vi "10-2.vi"() -> ()   [LabVIEW 2022 SP3, in "AoC22.lvlib"]
uses:
  AoC22.lvlib
  <vilib>/IlluminatedG/lv-stream/Stream.lvlib
panel:
  out "Array":bool[][](array[boolean])
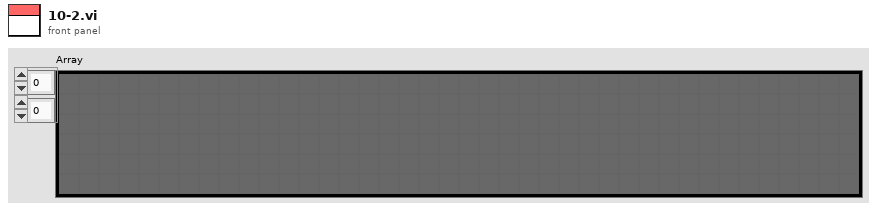
[diagram p1: front panel]
types:
  T1 = cluster{"String":string, "String":string, "x":i32, i32, i32, bool}
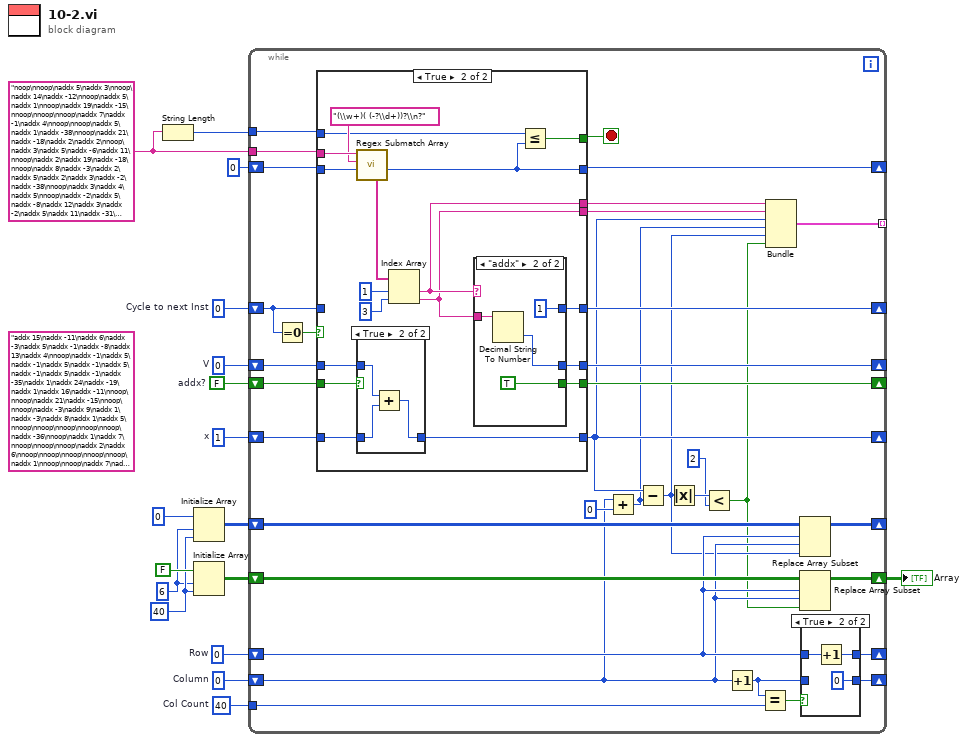
[diagram p0: block diagram]
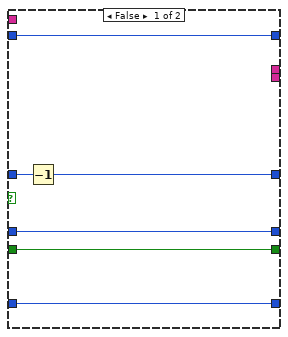
[diagram p3: hidden frame]
diagram:
  w4 = 40 ("dimension size")
  w3 = 6 ("dimension size")
  w9 = 0  # Row
  (unwired) "addx 15\naddx -11\naddx 6\naddx -3\naddx 5\naddx -1\naddx -8\naddx 13\naddx 4\nnoop\naddx -1\naddx 5\naddx -1\naddx 5\naddx -1\naddx 5\naddx -1\naddx 5\naddx -1\naddx -35\naddx 1\naddx 24\naddx -19\naddx 1\naddx 16\naddx -11\nnoop\nnoop\naddx 21\naddx -15\nnoop\nnoop\naddx -3\naddx 9\naddx 1\naddx -3\naddx 8\naddx 1\naddx 5\nnoop\nnoop\nnoop\nnoop\nnoop\naddx -36\nnoop\naddx 1\naddx 7\nnoop\nnoop\nnoop\naddx 2\naddx 6\nnoop\nnoop\nnoop\nnoop\nnoop\naddx 1\nnoop\nnoop\naddx 7\naddx 1\nnoop\naddx -13\naddx 13\naddx 7\nnoop\naddx 1\naddx -33\nnoop\nnoop\nnoop\naddx 2\nnoop\nnoop\nnoop\naddx 8\nnoop\naddx -1\naddx 2\naddx 1\nnoop\naddx 17\naddx -9\naddx 1\naddx 1\naddx -3\naddx 11\nnoop\nnoop\naddx 1\nnoop\naddx 1\nnoop\nnoop\naddx -13\naddx -19\naddx 1\naddx 3\naddx 26\naddx -30\naddx 12\naddx -1\naddx 3\naddx 1\nnoop\nnoop\nnoop\naddx -9\naddx 18\naddx 1\naddx 2\nnoop\nnoop\naddx 9\nnoop\nnoop\nnoop\naddx -1\naddx 2\naddx -37\naddx 1\naddx 3\nnoop\naddx 15\naddx -21\naddx 22\naddx -6\naddx 1\nnoop\naddx 2\naddx 1\nnoop\naddx -10\nnoop\nnoop\naddx 20\naddx 1\naddx 2\naddx 2\naddx -6\naddx -11\nnoop\nnoop\nnoop"
  w11 = 40  # Col Count
  w12 = 0  # Column
  w13 = FALSE  # addx?
  w15 = 1  # x
  w14 = 0  # V
  w16 = 0  # Cycle to next Inst
  w1 = "noop\nnoop\naddx 5\naddx 3\nnoop\naddx 14\naddx -12\nnoop\naddx 5\naddx 1\nnoop\naddx 19\naddx -15\nnoop\nnoop\nnoop\naddx 7\naddx -1\naddx 4\nnoop\nnoop\naddx 5\naddx 1\naddx -38\nnoop\naddx 21\naddx -18\naddx 2\naddx 2\nnoop\naddx 3\naddx 5\naddx -6\naddx 11\nnoop\naddx 2\naddx 19\naddx -18\nnoop\naddx 8\naddx -3\naddx 2\naddx 5\naddx 2\naddx 3\naddx -2\naddx -38\nnoop\naddx 3\naddx 4\naddx 5\nnoop\naddx -2\naddx 5\naddx -8\naddx 12\naddx 3\naddx -2\naddx 5\naddx 11\naddx -31\naddx 23\naddx 4\nnoop\nnoop\naddx 5\naddx 3\naddx -2\naddx -37\naddx 1\naddx 5\naddx 2\naddx 12\naddx -10\naddx 3\naddx 4\naddx -2\nnoop\naddx 6\naddx 1\nnoop\nnoop\nnoop\naddx -2\naddx 7\naddx 2\nnoop\naddx 3\naddx 3\naddx 1\nnoop\naddx -37\naddx 2\naddx 5\naddx 2\naddx 32\naddx -31\naddx 5\naddx 2\naddx 9\naddx 9\naddx -15\nnoop\naddx 3\naddx 2\naddx 5\naddx 2\naddx 3\naddx -2\naddx 2\naddx 2\naddx -37\naddx 5\naddx -2\naddx 2\naddx 5\naddx 2\naddx 16\naddx -15\naddx 4\nnoop\naddx 1\naddx 2\nnoop\naddx 3\naddx 5\naddx -1\naddx 5\nnoop\nnoop\nnoop\nnoop\naddx 3\naddx 5\naddx -16\nnoop"
  n1 = String Length(string=w1) -> (length=w17:i32)
  n2 = Initialize Array(0, w3, w4) -> (w2:i32[][])
  n3 = Initialize Array(FALSE, w3, w4) -> (w7:bool[][])
  n4 = while {
    tunnel: w1 -> [w51]
    shift-right: [w48] -> _
    shift-left: 0 ("offset past match") -> [w50]
    tunnel: w17 -> [w49]
    shift-right: [w42] -> _
    shift-left: w16 -> [w45]
    shift-right: [w23] -> _
    shift-left: w15 -> [w27]
    shift-right: [w41] -> _
    shift-left: w14 -> [w44]
    shift-right: [w40] -> _
    shift-left: w13 -> [w43]
    shift-right: [w36] -> _
    shift-left: w12 -> [w22]
    tunnel: w11 -> [w39]
    shift-right: [w35] -> _
    shift-left: w9 -> [w28]
    shift-right: [w31] -> w6
    shift-left: w7 -> [w32]
    shift-right: [w30] -> _
    shift-left: w2 -> [w29]
    tunnel: [w19] -> _ mode=indexing
    stop <- w47 stop-if-true
    n5 = Equal To 0?(x=w45) -> (x = 0?=w46:bool)
    n6 = case shown="True" w46 {
      tunnel: w51 -> [_ w80]
      tunnel: w50 -> [w58 w78]
      tunnel: w49 -> [_ w77]
      tunnel: [w58 w66] -> w48
      tunnel: [_ w76] -> w47
      tunnel: w45 -> [w62 _]
      tunnel: w44 -> [w60 w70]
      tunnel: w27 -> [w57 w71]
      tunnel: w43 -> [w59 w72]
      tunnel: [w61 w67] -> w42
      tunnel: [w57 w65] -> w23
      tunnel: [w60 w69] -> w41
      tunnel: [w59 w68] -> w40
      tunnel: [_ w64] -> w25
      tunnel: [_ w63] -> w24
      frame False {
        n7 = Decrement(x=w62) -> (x-1=w61:i32)
      }
      frame True {
        n8 = call <vilib>:"Regex Submatch Array.vi"("offset (0)"=w78, "regular expression"="(\\w+)( (-?\\d+))?\\n?", "string"=w80) -> ("offset past match"=w66:i32, "matches"=w75:string[])  [unwired: 6 in, 1 out]
        n9 = case shown="True" w72 {
          tunnel: w71 -> [w81 w84]
          tunnel: w70 -> [_ w83]
          tunnel: [w81 w82] -> w65
          frame False {
          }
          frame True {
            n10 = Add(x=w83, y=w84) -> (x+y=w82:i32)
          }
        }
        n11 = Index Array(array=w75, index #1=1 ("index"), index #2=3 ("index")) -> (element #1=w64:string, element #2=w63:string)
        n12 = case shown="\"addx\"" w64 {
          tunnel: w63 -> [_ w88]
          tunnel: [_ w87] -> w69
          tunnel: [_ TRUE] -> w68
          tunnel: [_ 1] -> w67
          frame "noop", Default {
          }
          frame "addx" {
            n13 = Decimal String To Number(string=w88) -> (number=w87:i32)  [unwired: 2 in, 1 out]
          }
        }
        n14 = Less Or Equal?(x=w77, y=w66) -> (x <= y?=w76:bool)
      }
    }
    n15 = Add(x=w22, y=0) -> (x+y=w18:i32)
    n16 = Subtract(x=w23, y=w18) -> (x-y=w21:i32)
    n17 = Absolute Value(x=w21) -> (abs(x)=w34:i32)
    n18 = Less?(x=w34, y=2) -> (x < y?=w20:bool)
    n19 = Increment(x=w22) -> (x+1=w37:i32)
    n20 = Equal?(x=w37, y=w39) -> (x = y?=w38:bool)
    n21 = Bundle("String"=w25, "String"=w24, "x"=w23, w18, w21, w20) -> (w19:T1)  [unwired: 1 in]
    n22 = Replace Array Subset(array=w29, new element=w21, index (row)=w28, index (col)=w22) -> (w30:i32[][])
    n23 = Replace Array Subset(array=w32, new element=w20, index (row)=w28, index (col)=w22) -> (w31:bool[][])
    n24 = case shown="True" w38 {
      tunnel: w28 -> [w52 w56]
      tunnel: w37 -> [w53 _]
      tunnel: [w53 0] -> w36
      tunnel: [w52 w55] -> w35
      frame False {
      }
      frame True {
        n25 = Increment(x=w56) -> (x+1=w55:i32)
      }
    }
  }
  "Array" <- w6
